vi "Folder Packaging.vi"() -> ()   [LabVIEW 2019, in "NIPM Packaging.lvlib"]
uses:
  NIPM Packaging.lvlib
  <vilib>/National Instruments/NIPM API (Beta)/NIPM_API.lvlib
panel:
  out "error out":errorcluster
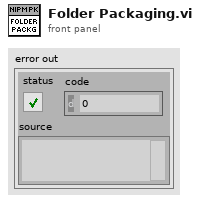
[diagram p1: front panel]
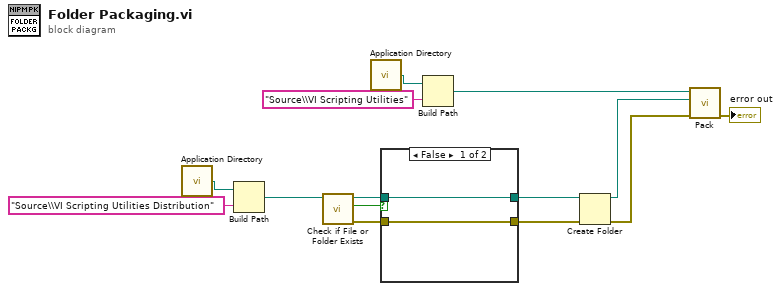
[diagram p0: block diagram]
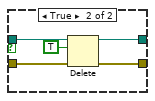
[diagram p2: hidden frame]
diagram:
  n1 = call <vilib>:"Application Directory.vi"() -> ("Application Directory"=w10:path)
  n2 = Build Path(base path=w10, name or relative path="Source\\VI Scripting Utilities Distribution") -> (appended path=w9:path)
  n3 = call <vilib>:"Check if File or Folder Exists.vi"("path"=w9) -> ("error out"=w6:errorcluster, "file or folder exists?"=w8:bool, "dup path"=w7:path)  [unwired: 8 in]
  n4 = call <vilib>:"Application Directory.vi"() -> ("Application Directory"=w14:path)
  n5 = case shown="False" w8 {
    tunnel: w7 -> [w16 w21]
    tunnel: w6 -> [w15 w20]
    tunnel: [w16 w18] -> w4
    tunnel: [w15 w17] -> w5
    frame False {
    }
    frame True {
      n6 = Delete(path (use dialog)=w21, entire hierarchy (F)=TRUE, error in=w20) -> (deleted path=w18:path, error out=w17:errorcluster)  [unwired: 2 in, 1 out]
    }
  }
  n7 = Build Path(base path=w14, name or relative path="Source\\VI Scripting Utilities") -> (appended path=w12:path)
  n8 = Create Folder(path (use dialog)=w4, error in=w5) -> (created path=w3:path, error out=w2:errorcluster)  [unwired: 1 in, 1 out]
  n9 = call <vilib>:"Pack.vi"("error in"=w2, "destination folder"=w3, "source folder"=w12) -> ("error out"=→"error out":errorcluster)  [unwired: 7 in, 1 out]
